vi "Search Integer Array for Negatives.vi"(11 "JSON Parser in":refnum<class "JSON Parser.lvclass">) -> (1 "Current Array is Signed Integer?":bool, 2 "Search Integer Array for Negatives?":bool, 3 "JSON Parser out":refnum<class "JSON Parser.lvclass">, 5 "Currently Parsing an Array?":bool)   [LabVIEW 2020, in "JKI JSON Serialization.lvlib" / "JSON Parser.lvclass"]
uses:
  JSON Parser.lvclass
  JSON Parser.lvclass/JSON Parser.ctl
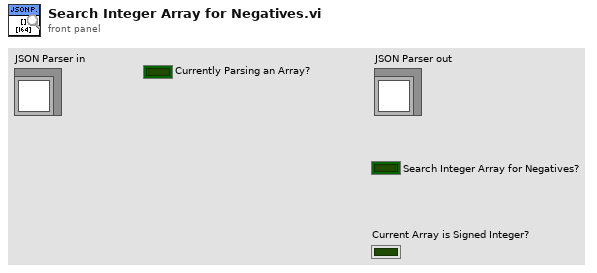
[diagram p1: front panel]
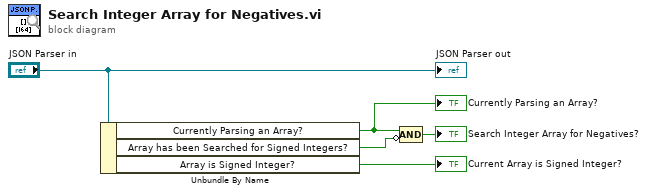
[diagram p0: block diagram]
diagram:
  n1 = Unbundle By Name("JSON Parser in") -> ("Currently Parsing an Array?"=w5:bool, "Array has been Searched for Signed Integers?"=w1:bool, "Array is Signed Integer?"=→"Current Array is Signed Integer?":bool)
  "Currently Parsing an Array?" <- w5
  n2 = Compound Arithmetic op=AND(w5, invert w1) -> (→"Search Integer Array for Negatives?":bool)
  "JSON Parser out" <- "JSON Parser in"
